vi "spietro_savechanges.vi"() -> ()   [LabVIEW 2010]
uses:
  <vilib>/Utility/file.llb/Write To Spreadsheet File (I64).vi
panel:
  in  "Data file path ending":string=".dat"
  out "date/time string":string
  in  "time format string (%c)":string="%Y-%m-%d %H-%M.%S"
  in  "Auto Save Data?":bool
  out "Previous Acquisition":u16[](graph)
  out "Current Acquisition":u16[](graph)
  out "ErrCode":i32
  out "ErrMsg":string
  in  "InterChannel Delay":sgl=-1.0 format="%.2f"
  in  "LowChan":i32
  in  "HighChan":i32
  in  "Options":i32
  in  "Range":i32(ring)=2 items=["Not Programmable"=0, "+- 20 V"=27, "+- 10 V"=1, "+- 5 V"=2, "+- 4 V"=28, "+- 2.5 V"=3, "+- 2 V"=29, "+- 1.67 V"=4, "+- 1.25 V"=5, "+- 1 V"=6, "+- .625 V"=7, "+- .5 V"=8, "+- .25 V"=30, "+- .2 V"=31, "+- .1 V"=9, "+- .05 V"=10, "+- .01 V"=11, "+- .005 V"=12, "0 - 10 V"=13, "0 - 5 V"=14, "0 - 4 V"=36, "0 - 2.5 V"=15, "0 - 2 V"=16, "0 - 1.67 V"=17, "0 - 1.25 V"=18, "0 - 1 V"=19, "0 - .5 V"=32, "0 - .25 V"=33, "0 - .2 V"=34, "0 - .1 V"=20, "0 - .02 V"=35, "0 - .01 V"=21, "4 - 20 mA"=22, "2 - 10 mA"=23, "1 - 5 mA"=24, ".5 - 2.5 mA"=25, "0 - 20 mA"=26]
  in  "Rate":i32
  in  "Count":i32
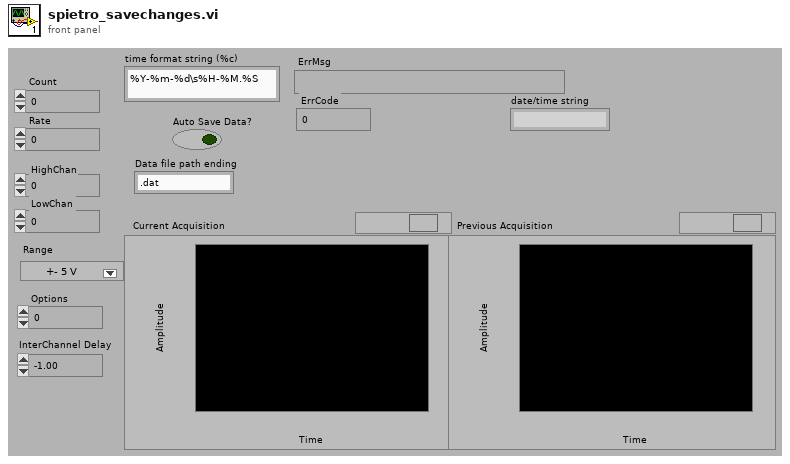
[diagram p1: front panel]
types:
  T1 = typedef "imagedata.ctl" = cluster{"image type":i32, "image depth":i32, "image":u8[], "mask":u8[], "colors":u32[], "Rectangle":cluster{"left":i16, "top":i16, "right":i16, "bottom":i16}}
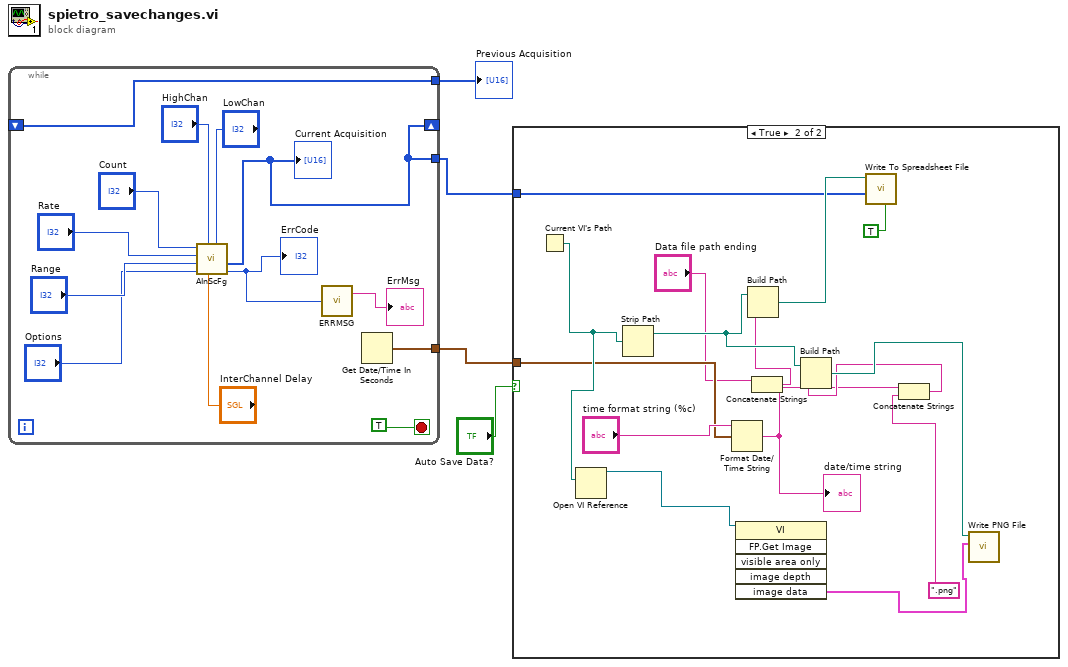
[diagram p0: block diagram]
diagram:
  n1 = while {
    shift-right: [w5] -> _
    shift-left: _ -> [w7]
    tunnel: [w7] -> w4
    tunnel: [w6] -> w2
    tunnel: [w5] -> w1
    stop <- TRUE stop-if-true
    n2 = call <menus>:"AInScFg.VI"("LowChan"="LowChan", "InterChannel Delay"="InterChannel Delay", "HighChan"="HighChan", "Options"="Options", "Range"="Range", "Rate"="Rate", "Count"="Count") -> ("ErrCode"=w9:i32, "ADData"=w5:u16[])  [unwired: 1 in, 1 out]
    "ErrCode" <- w9
    "Current Acquisition" <- w5
    n3 = call <menus>:"ERRMSG.VI"("ErrCode"=w9) -> ("ErrMsg"=→"ErrMsg":string)  [unwired: 1 out]
    n4 = Get Date/Time In Seconds() -> (seconds since 1Jan1904=w6:timestamp)
  }
  "Previous Acquisition" <- w4
  n5 = case shown="True" "Auto Save Data?" {
    tunnel: w2 -> [_ w25]
    tunnel: w1 -> [_ w21]
    frame False {
    }
    frame True {
      n6 = Current VI's Path() -> (path=w32:path)
      n7 = Open VI Reference(vi path=w32) -> (vi reference=w20:refnum<vi>)  [unwired: 5 in, 1 out]
      n8 = Strip Path(path=w32) -> (stripped path=w30:path)  [unwired: 1 out]
      n9 = Format Date/Time String(time format string (%c)="time format string (%c)", seconds (now)=w25) -> (date/time string=w22:string)  [unwired: 1 in]
      "date/time string" <- w22
      n10 = invoke class="VI" method="FP.Get Image"(reference=w20) -> ("image data"=w18:T1)  [unwired: 5 in, 5 out]
      n11 = Concatenate Strings("Data file path ending", w22) -> (w23:string)
      n12 = Build Path(base path=w30, name or relative path=w23) -> (appended path=w28:path)
      n13 = call-poly <vilib>:"Write To Spreadsheet File.vi"("transpose? (no:F)"=TRUE, "1D data"=w21, "file path (dialog if empty)"=w28) -> ()  [unwired: 5 in, 1 out]
      n14 = Concatenate Strings(w22, ".png" ("string")) -> (w26:string)
      n15 = Build Path(base path=w30, name or relative path=w26) -> (appended path=w29:path)
      n16 = call <vilib>:"Write PNG File.vi"("image data"=w18, "path to PNG file"=w29) -> ()  [unwired: 8 in, 2 out]
    }
  }
